vi "TDT-Stream AI.vi"(0 "RPcox":refnum<k7>, 2 "Action":T1=enum."Read", 7 "Pts Per Read":i32, 9 "AI only":bool, 11 "error in (no error)":errorcluster, 12 "AI Channels":i32[](array[numeric])=[1, 2]) -> (4 "RPcoX thru":refnum<k7>, 10 "AI Waveforms":dbl[][](array[numeric]), 15 "error out":errorcluster)   [LabVIEW 2020]
uses:
  TDT-Signal Bank Action.ctl
  TDT-Globals.vi
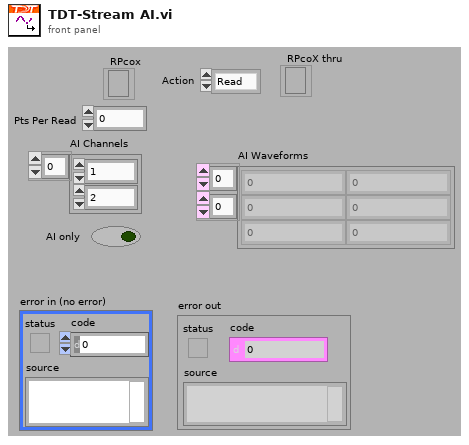
[diagram p1: front panel]
types:
  T1 = typedef "TDT-Signal Bank Action.ctl" = enum16{"Init", "Write", "Read", "Rewrite", "Reset", "Recycle", "Ramp up", "Ramp down", "Zero"}
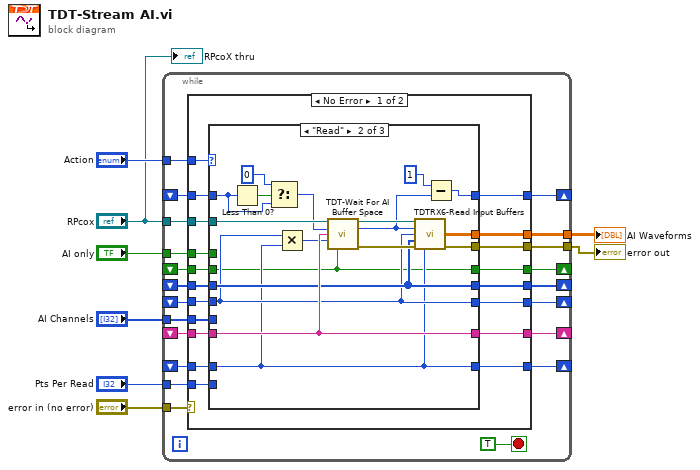
[diagram p0: block diagram]
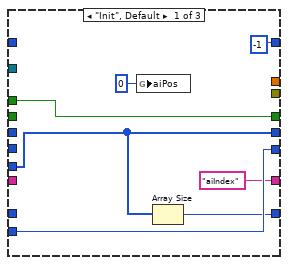
[diagram p2: hidden frame]
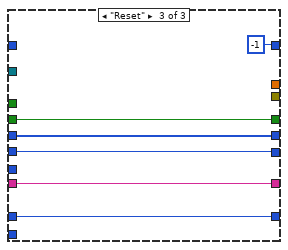
[diagram p3: hidden frame]
diagram:
  n1 = while {
    tunnel: [w29] -> w7
    tunnel: "error in (no error)" -> [w28]
    tunnel: "RPcox" -> [w27]
    tunnel: "Action" -> [w26]
    shift-right: [w24] -> _
    shift-left: _ -> [w23]
    tunnel: "Pts Per Read" -> [w22]
    shift-right: [w21] -> _
    shift-left: _ -> [w20]
    tunnel: [w19] -> w4
    tunnel: "AI Channels" -> [w18]
    shift-right: [w17] -> _
    shift-left: _ -> [w16]
    shift-right: [w15] -> _
    shift-left: _ -> [w14]
    shift-right: [w12] -> _
    shift-left: _ -> [w13]
    shift-right: [w10] -> _
    shift-left: _ -> [w11]
    tunnel: "AI only" -> [w9]
    stop <- TRUE stop-if-true
    n2 = case shown="No Error" w28 {
      selector: w28 -> [_ w86]
      tunnel: [w44 w86] -> w29
      tunnel: w27 -> [w45 _]
      tunnel: w26 -> [w48 _]
      tunnel: [w47 w85] -> w24
      tunnel: w23 -> [w46 w85]
      tunnel: w22 -> [w43 _]
      tunnel: [w42 w84] -> w21
      tunnel: w20 -> [w41 w84]
      tunnel: [w40 _] -> w19
      tunnel: w18 -> [w39 _]
      tunnel: [w38 w83] -> w17
      tunnel: w16 -> [w37 w83]
      tunnel: [w36 w82] -> w15
      tunnel: w14 -> [w35 w82]
      tunnel: w13 -> [w34 w81]
      tunnel: [w33 w81] -> w12
      tunnel: w11 -> [w32 w80]
      tunnel: [w31 w80] -> w10
      tunnel: w9 -> [w30 _]
      frame No Error {
        n3 = case shown="\"Read\"" w48 {
          tunnel: [-1 w73 -1] -> w47
          tunnel: w46 -> [_ w64 _]
          tunnel: w45 -> [_ w70 _]
          tunnel: [_ w68 _] -> w44
          tunnel: w43 -> [w54 _ _]
          tunnel: [w54 w58 w78] -> w42
          tunnel: w41 -> [_ w58 w78]
          tunnel: [_ w66 _] -> w40
          tunnel: w39 -> [w49 _ _]
          tunnel: [w49 w59 w79] -> w38
          tunnel: w37 -> [_ w59 w79]
          tunnel: ["aiIndex" ("format string") w61 w77] -> w36
          tunnel: w35 -> [_ w61 w77]
          tunnel: w34 -> [_ w57 w75]
          tunnel: [w50 w57 w75] -> w33
          tunnel: w32 -> [_ w56 w74]
          tunnel: [w51 w56 w74] -> w31
          tunnel: w30 -> [w51 _ _]
          frame "Init", Default {
            n4 = global write "TDT-Globals.vi" "aiPos"(0 ("aiPos")) -> ()
            n5 = Array Size(array=w49) -> (size(s)=w50:i32)
          }
          frame "Read" {
            n6 = Less Than 0?(x=w64) -> (x < 0?=w65:bool)
            n7 = Select(t=0, s=w65, f=w64) -> (s? t:f=w62:i32)
            n8 = Multiply(x=w58, y=w57) -> (x*y=w60:i32)
            n9 = call "TDT-Wait For AI Buffer Space.vi"("RPcox"=w70, "Next Buffer"=w62, "Tag"=w61, "Buffer Length"=w60, "AI only"=w56) -> ("RPcox Out"=w69:refnum<k7>, "Next Buffer Out"=w67:i32, "error out"=w71:errorcluster)  [unwired: 8 in]
            n10 = call "TDTRX6-Read Input Buffers.vi"("RPcox"=w69, "Next Buffer"=w67, "Pts Per Read"=w58, "AI Channels"=w59, "error in (no error)"=w71, "#inputs"=w57) -> ("Input array"=w66:dbl[][], "error out"=w68:errorcluster)  [unwired: 8 in]
            n11 = Subtract(x=1, y=w67) -> (x-y=w73:i32)
          }
          frame "Reset" {
          }
        }
      }
      frame Error {
      }
    }
  }
  "error out" <- w7
  "AI Waveforms" <- w4
  "RPcoX thru" <- "RPcox"
